vi "Close.vi"(8 "error in (no error)":errorcluster caption="Fehler (Eingang, kein Fehler)", 11 "Data IN":T1) -> (0 "error out":errorcluster caption="Fehler (Ausgang)", 3 "Data Out":T1)   [LabVIEW 2020, in "Hardware A.lvlib"]
uses:
  Hardware A.lvlib
  Data.ctl
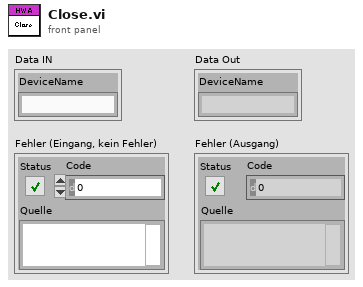
[diagram p1: front panel]
types:
  T1 = typedef "Hardware A.lvlib/Data.ctl" = cluster{"DeviceName":string}
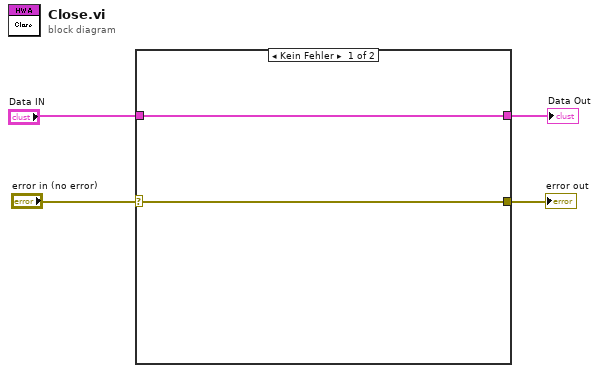
[diagram p0: block diagram]
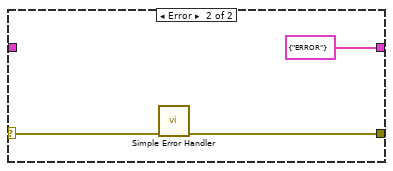
[diagram p2: hidden frame]
diagram:
  n1 = case shown="Kein Fehler" "error in (no error)" {
    selector: "error in (no error)" -> [w6 w9]
    tunnel: [w6 w8] -> w3
    tunnel: "Data IN" -> [w5 _]
    tunnel: [w5 cluster{"DeviceName":string} {"DeviceName"="ERROR"} ("Data IN")] -> w1
    frame No Error {
    }
    frame Error {
      n2 = call <vilib>:"Simple Error Handler.vi"("error in (no error)"=w9) -> ("error out"=w8:errorcluster)  [unwired: 4 in, 4 out]
    }
  }
  "error out" <- w3
  "Data Out" <- w1
